vi "Launch Helper Loop.vi"(8 "error in (no error)":errorcluster, 9 "Message Data":variant, 10 "Message":string, 11 "Helper Loop In":refnum<class "Helper Loop.lvclass">) -> (0 "error out":errorcluster, 3 "Helper Loop Out":refnum<class "Helper Loop.lvclass">)   [LabVIEW 2020, in "Helper Loop.lvclass"]
doc: "Launches an asynchronous helper loop. Multiple helper loops may be launched using multiple calls to this VI. The Message and Message Data provided to this VI will be available in the Helper Action.vi once running."
uses:
  Helper Loop.lvclass
  <vilib>/Utility/error.llb/Error Cluster From Error Code.vi
  <vilib>/ErrorRing/Error Ring.xnode
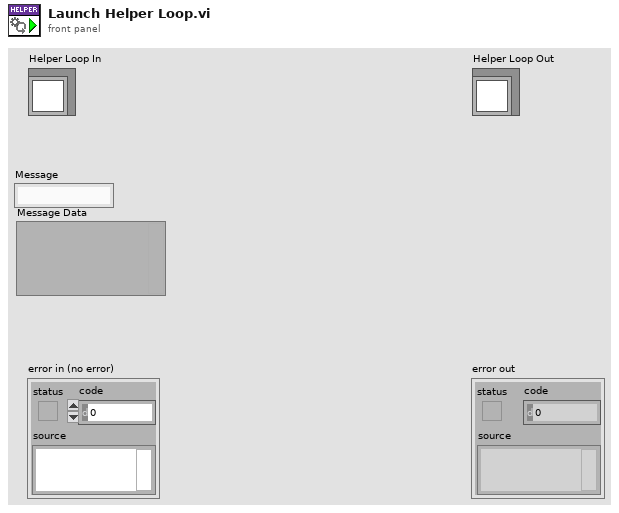
[diagram p1: front panel]
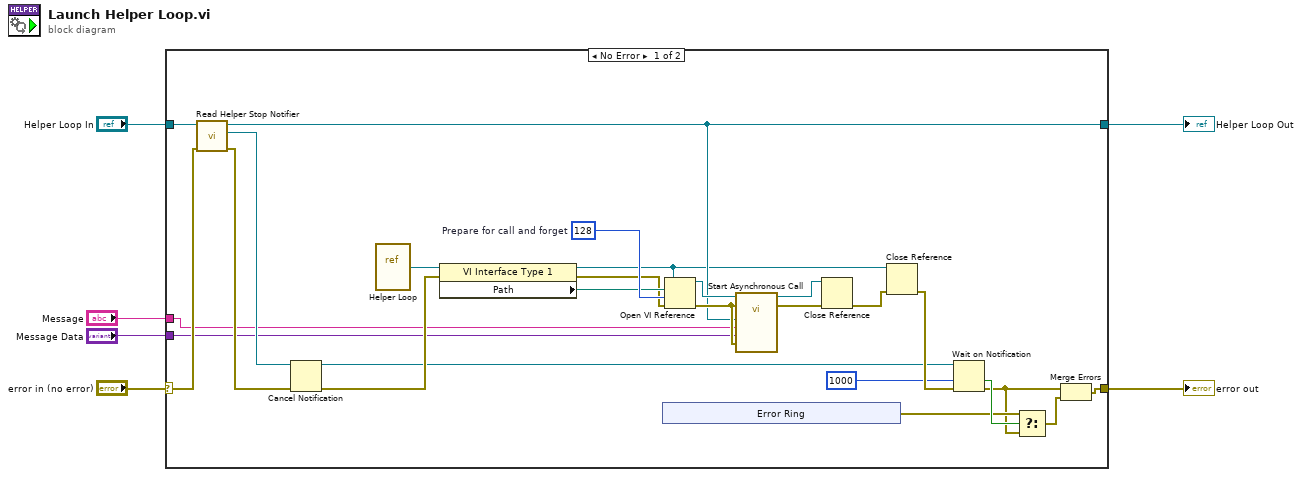
[diagram p0: block diagram]
diagram:
  n1 = case shown="No Error" "error in (no error)" {
    selector: "error in (no error)" -> [w20 w38]
    tunnel: [w9 w38] -> w5
    tunnel: [w21 w37] -> w4
    tunnel: "Helper Loop In" -> [w22 w37]
    tunnel: "Message" -> [w16 _]
    tunnel: "Message Data" -> [w15 _]
    frame No Error {
      w29 = 128  # Prepare for call and forget
      n2 = call-dynamic "Read Helper Stop Notifier.vi"("error in (no error)"=w20, "Helper Loop In"=w22) -> ("error out"=w19:errorcluster, "Helper Stopped Notifier"=w17:refnum<notifier>, "Helper Loop Out"=w21:refnum<class "Helper Loop.lvclass">)  [unwired: 7 in]
      n3 = Cancel Notification(0:w17, 3:w19) -> (8:w14:refnum<notifier>, 11:w18:errorcluster)  [unwired: 1 out]
      n4 = vi-ref "Helper Loop.vi"() -> (w30:refnum<vi>)
      n5 = property class="VI Interface Type 1"(reference=w30, error in=w18) -> (reference out=w7:refnum<vi>, error out=w25:errorcluster, "Path"=w27:path)
      n6 = xnode "Error Ring"() -> ("error out"=w11:errorcluster)
      n7 = Open VI Reference(type specifier VI Refnum (for type only)=w7, vi path=w27, options=w29, error in (no error)=w25) -> (vi reference=w28:refnum<vi>, error out=w26:errorcluster)  [unwired: 2 in]
      n8 = call-by-ref "Start Asynchronous Call"(reference=w28, error in=w26, 8:"error in (no error)"=w26, "Message Data"=w15, "Message"=w16, "Helper Loop In"=w21) -> (reference out=w32:refnum<vi>, error out=w31:errorcluster)  [unwired: 6 in, 2 out]
      n9 = Close Reference(reference=w32, error in (no error)=w31) -> (error out=w24:errorcluster)
      n10 = Close Reference(reference=w7, error in (no error)=w24) -> (error out=w23:errorcluster)
      n11 = Wait on Notification(notifier=w14, timeout in ms (-1)=1000, error in (no error)=w23) -> (timed out?=w12:bool, error out=w10:errorcluster)  [unwired: 1 in, 2 out]
      n12 = Select(t=w11, s=w12, f=w10) -> (s? t:f=w8:errorcluster)
      n13 = Merge Errors(w10, w8) -> (w9:errorcluster)
    }
    frame Error {
    }
  }
  "error out" <- w5
  "Helper Loop Out" <- w4
